vi "Calculate FPS Microsoft Camera.vi"() -> (2 "Fps":dbl)   [LabVIEW 2019]
uses:
  <vilib>/ptbypt/NI_PtbyPt.lvlib
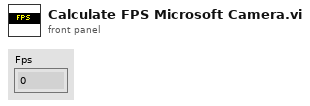
[diagram p1: front panel]
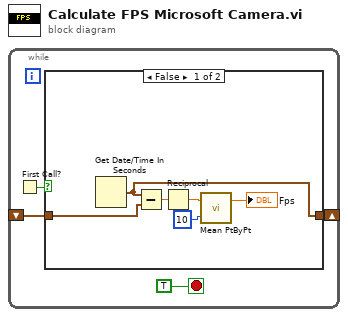
[diagram p0: block diagram]
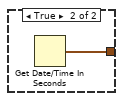
[diagram p2: hidden frame]
diagram:
  n1 = while {
    shift-right: [w3] -> _
    shift-left: _ -> [w4]
    stop <- TRUE stop-if-true
    n2 = First Call?() -> (First Call?: T/F=w1:bool)
    n3 = case shown="False" w1 {
      tunnel: w4 -> [w10 _]
      tunnel: [w9 w11] -> w3
      frame False {
        n4 = Get Date/Time In Seconds() -> (seconds since 1Jan1904=w9:timestamp)
        n5 = Subtract(x=w9, y=w10) -> (x-y=w7:dbl)
        n6 = Reciprocal(x=w7) -> (1/x=w8:dbl)
        n7 = call <vilib>:"Mean PtByPt.vi"("x"=w8, "sample length"=10) -> ("mean"=→"Fps":dbl)  [unwired: 2 in, 1 out]
      }
      frame True {
        n8 = Get Date/Time In Seconds() -> (seconds since 1Jan1904=w11:timestamp)
      }
    }
  }
